vi "waitForMeasureReady.vi"(0 "drv":u32) -> ()   [LabVIEW 2015]
uses:
  ESLSCDLL.dll
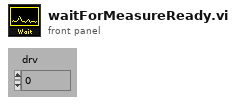
[diagram p1: front panel]
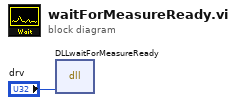
[diagram p0: block diagram]
diagram:
  n1 = dll-call lib="C:/ENTW/PCIE/lv64/board.vis/ESLSCDLL.dll" fn="DLLwaitForMeasureReady" ("lwlscdll.dll:DLLWriteLongS0")("drv"="drv") -> ()  [unwired: 5 in, 2 out]
